vi "SLSC Load EDS Configuration.vi"(0 "selected path":path, 11 "error in (no error)":errorcluster) -> (1 "Type of file":i32(ring) items=["Not a Valid File", "SLSC Capability File", "SLSC EDS Configuration"], 3 "Loop rate":u32, 4 "SLSC EDS module out":T2, 6 "Enable Channels":string[](array[string]), 8 "Custom Device Name":string, 10 "Has capability?":bool, 12 "Apply Default":bool, 13 "Custom Device Description":string, 14 "Apply Reset":bool, 15 "error out":errorcluster)   [LabVIEW 2020, in "SLSC EDS System Explorer.lvlib"]
uses:
  System Explorer/SLSC EDS System Explorer.lvlib
  SLSC EDS API/JSON parsing/EDSjsonStructure.ctl
  SLSC EDS API/JSON parsing/enum.ctl
  SLSC EDS API/JSON parsing/property.ctl
  SLSC EDS API/JSON parsing/command.ctl
  SLSC EDS API/JSON parsing/scale.ctl
  SLSC EDS API/JSON parsing/physicalChannel.ctl
  SLSC EDS API/JSON parsing/register.ctl
  SLSC EDS API/JSON parsing/EDS_Custom_Device_Structure.ctl
  <vilib>/addons/_JKI.lib/Serialization/JSON/JKI JSON Serialization.lvlib
panel:
  out "text":string
  in  "Value":T1
  # "not working\nregisterMap->registers->initialValue"
  # "not working\nregisterMap->registers->initialValue"
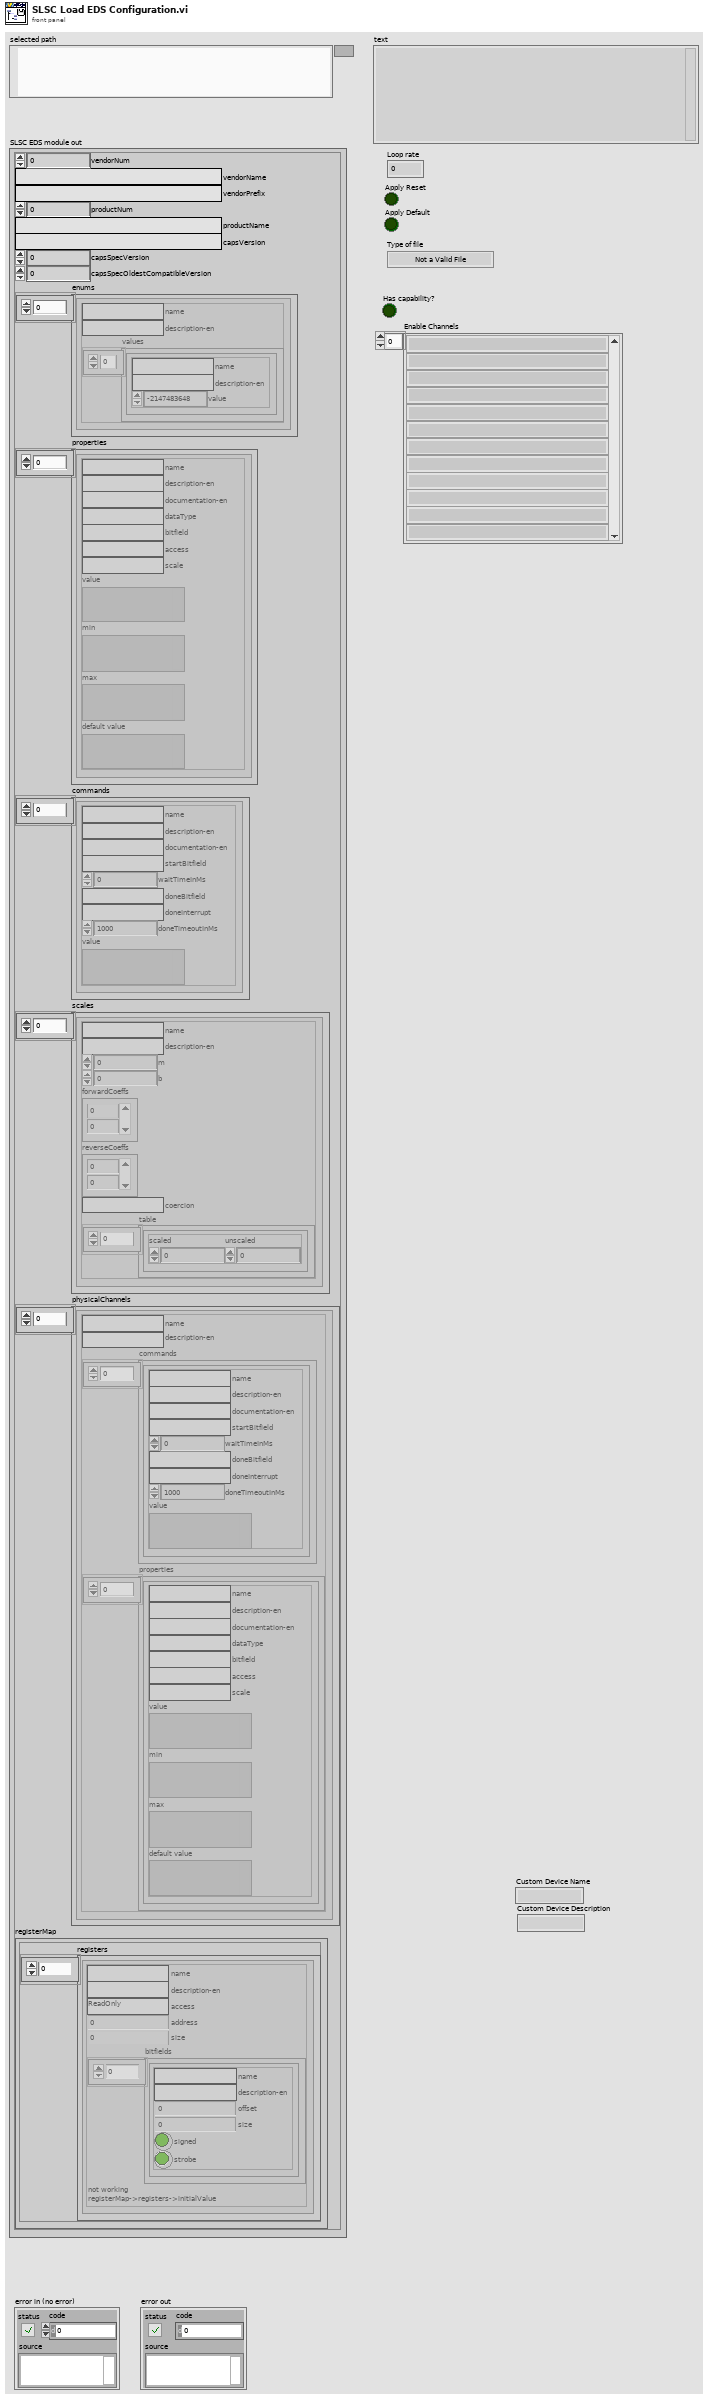
[diagram p1: front panel]
types:
  T1 = typedef "EDS_Custom_Device_Structure.ctl" = cluster{"SLSC EDS module out":T2, "Custom Device Name":string, "TreeItem Channels":string[], "Apply Default":bool, "Apply Reset":bool, "Loop rate":u32, "Custom Device Description":string}
  T2 = typedef "EDSjsonStructure.ctl" = cluster{"vendorNum":u32, "vendorName":string, "vendorPrefix":string, "productNum":u32, "productName":string, "capsVersion":string, "capsSpecVersion":u32, "capsSpecOldestCompatibleVersion":u32, "enums":T3[], "properties":T4[], "commands":T5[], "scales":T6[], "physicalChannels":T7[], "registerMap":cluster{"registers":T8[]}}
  T3 = typedef "enum.ctl" = cluster{"name":string, "description-en":string, "values":cluster{"name":string, "description-en":string, "value":i32}[]}
  T4 = typedef "property.ctl" = cluster{"name":string, "description-en":string, "documentation-en":string, "dataType":string, "bitfield":string, "access":string, "scale":string, "value":variant, "min":variant, "max":variant, "default value":variant}
  T5 = typedef "command.ctl" = cluster{"name":string, "description-en":string, "documentation-en":string, "startBitfield":string, "waitTimeInMs":i32, "doneBitfield":string, "doneInterrupt":string, "doneTimeoutInMs":i32, "value":variant}
  T6 = typedef "scale.ctl" = cluster{"name":string, "description-en":string, "m":dbl, "b":dbl, "forwardCoeffs":dbl[], "reverseCoeffs":dbl[], "coercion":string, "table":cluster{"scaled":dbl, "unscaled":dbl}[]}
  T7 = typedef "physicalChannel.ctl" = cluster{"name":string, "description-en":string, "commands":T5[], "properties":T4[]}
  T8 = typedef "register.ctl" = cluster{"name":string, "description-en":string, "access":string, "address":u32, "size":u32, "bitfields":cluster{"name":string, "description-en":string, "offset":u32, "size":u32, "signed":bool, "strobe":bool}[]}
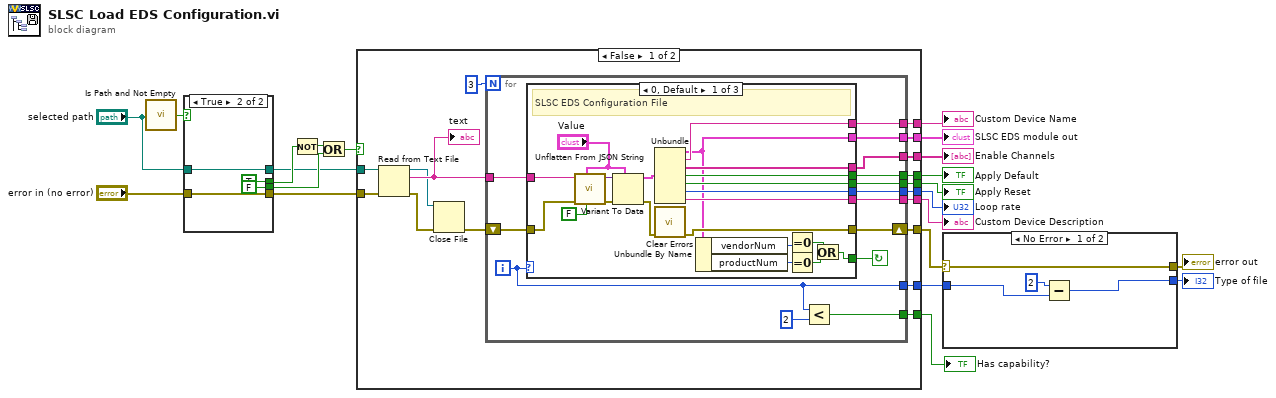
[diagram p0: block diagram]
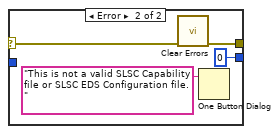
[diagram p2: hidden frame]
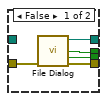
[diagram p3: hidden frame]
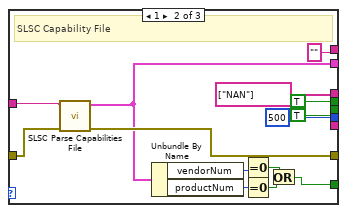
[diagram p4: hidden frame]
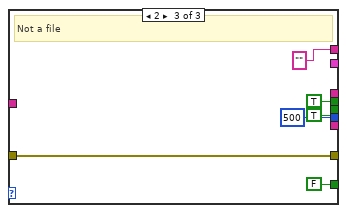
[diagram p5: hidden frame]
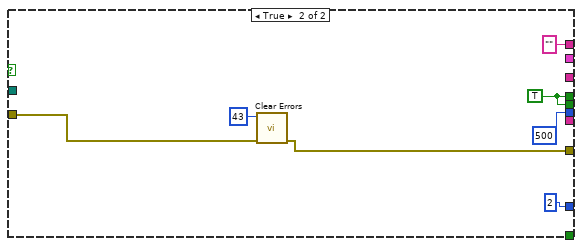
[diagram p6: hidden frame]
diagram:
  n1 = call <vilib>:"Is Path and Not Empty.vi"("path"="selected path") -> ("Is Path and Not Empty?"=w10:bool)  [unwired: 4 in]
  n2 = case shown="True" w10 {
    tunnel: [w26 TRUE ("exists")] -> w17
    tunnel: [w25 FALSE ("cancelled")] -> w15
    tunnel: "error in (no error)" -> [w24 w29]
    tunnel: [w23 w29] -> w13
    tunnel: [w22 w30] -> w12
    tunnel: "selected path" -> [_ w30]
    frame False {
      n3 = call "File Dialog"("error in"=w24) -> ("selected path"=w22:path, "exists"=w26:bool, "cancelled"=w25:bool, "error out"=w23:errorcluster)  [unwired: 11 in]
    }
    frame True {
    }
  }
  n4 = Not(x=w17) -> (.not. x?=w16:bool)
  n5 = Or(x=w16, y=w15) -> (x .or. y?=w11:bool)
  n6 = case shown="False" w11 {
    tunnel: [w47 _] -> w21
    tunnel: [w46 _] -> w20
    tunnel: [w44 w109] -> w2
    tunnel: [w43 w109] -> w1
    tunnel: [w42 u32 500 ("Loop rate")] -> w19
    tunnel: [w40 _] -> w18
    tunnel: [w39 w105] -> w8
    tunnel: w13 -> [w35 w106]
    tunnel: w12 -> [w34 _]
    tunnel: [w33 2] -> w6
    tunnel: [w32 "" ("Custom Device Name")] -> w4
    tunnel: [w31 _] -> w3
    frame False {
      n7 = Read from Text File(file (use dialog)=w34, error in=w35) -> (refnum out=w37:refnum<file>, text=w45:string, error out=w38:errorcluster)  [unwired: 2 in, 1 out]
      "text" <- w45
      n8 = Close File(refnum=w37, error in=w38) -> (error out=w36:errorcluster)  [unwired: 1 out]
      n9 = for {
        N: 3 -> [_]
        tunnel: [w60] -> w47
        tunnel: [w59] -> w46
        tunnel: w45 -> [w57]
        tunnel: [w56] -> w44
        tunnel: [w55] -> w43
        tunnel: [w54] -> w42
        shift-right: [w58] -> w39
        shift-left: w36 -> [w61]
        tunnel: [w51] -> w40
        tunnel: [w50] -> w33
        tunnel: [w49] -> w32
        tunnel: [w48] -> w31
        i -> [w50]
        stop <- w53 continue-if-true
        n10 = case shown="0, Default" w50 {
          tunnel: w61 -> [w82 w86 w99]
          tunnel: [w68 string[] ["NAN"] ("TreeItem Channels") _] -> w60
          tunnel: [w62 w84 _] -> w59
          tunnel: [w69 w85 w99] -> w58
          tunnel: w57 -> [w80 w87 _]
          tunnel: [w67 TRUE ("Apply Reset") TRUE ("Apply Reset")] -> w56
          tunnel: [w66 TRUE ("Apply Default") TRUE ("Apply Default")] -> w55
          tunnel: [w65 u32 500 ("Loop rate") u32 500 ("Loop rate")] -> w54
          tunnel: [w72 w89 FALSE] -> w53
          tunnel: [w63 "" ("Custom Device Name") "" ("Custom Device Name")] -> w49
          tunnel: [w64 _ _] -> w48
          frame 0, Default {
            # "SLSC EDS Configuration File"
            n11 = call <vilib>:"Unflatten From JSON String.vi"("Nulls as Defaults (F)"=FALSE, "Type and Defaults"="Value", "error in (no error)"=w82, "JSON String"=w80) -> ("error out"=w77:errorcluster, "Variant"=w78:variant)  [unwired: 6 in]
            n12 = Variant To Data(error in=w77, type="Value", Variant=w78) -> (data=w81:T1, error out=w70:errorcluster)
            n13 = Unbundle(w81) -> ("SLSC EDS module out"=w62:T2, "Custom Device Name"=w63:string, "TreeItem Channels"=w68:string[], "Apply Default"=w67:bool, "Apply Reset"=w66:bool, "Loop rate"=w65:u32, "Custom Device Description"=w64:string)
            n14 = call <vilib>:"Clear Errors.vi"("error in (no error)"=w70) -> ("error out"=w69:errorcluster)  [unwired: 5 in, 1 out]
            n15 = Unbundle By Name(w62) -> ("vendorNum"=w74:u32, "productNum"=w73:u32)
            n16 = Equal To 0?(x=w74) -> (x = 0?=w75:bool)
            n17 = Equal To 0?(x=w73) -> (x = 0?=w71:bool)
            n18 = Or(x=w75, y=w71) -> (x .or. y?=w72:bool)
          }
          frame 1 {
            # "SLSC Capability File"
            n19 = call "SLSC Parse Capabilities File.vi"("error in"=w86, "module capabilities JSON string"=w87) -> ("error out"=w85:errorcluster, "SLSC EDS module"=w84:T2)  [unwired: 7 in, 1 out]
            n20 = Unbundle By Name(w84) -> ("vendorNum"=w92:u32, "productNum"=w91:u32)
            n21 = Equal To 0?(x=w92) -> (x = 0?=w93:bool)
            n22 = Equal To 0?(x=w91) -> (x = 0?=w90:bool)
            n23 = Or(x=w93, y=w90) -> (x .or. y?=w89:bool)
          }
          frame 2 {
            # "Not a file"
          }
        }
        n24 = Less?(x=w50, y=2) -> (x < y?=w51:bool)
      }
    }
    frame True {
      w109 = TRUE ("Apply Reset")
      n25 = call <vilib>:"Clear Errors.vi"("error in (no error)"=w106, "specific error code to clear (0: all)"=43) -> ("error out"=w105:errorcluster)  [unwired: 4 in, 1 out]
    }
  }
  "Enable Channels" <- w21
  "SLSC EDS module out" <- w20
  "Apply Reset" <- w1
  "Apply Default" <- w2
  "Loop rate" <- w19
  "Has capability?" <- w18
  "Custom Device Name" <- w4
  "Custom Device Description" <- w3
  n26 = case shown="No Error" w8 {
    selector: w8 -> [w113 w115]
    tunnel: [w113 w116] -> w7
    tunnel: [w111 0] -> w5
    tunnel: w6 -> [w112 _]
    frame No Error {
      n27 = Subtract(x=2, y=w112) -> (x-y=w111:i32)
    }
    frame Error {
      n28 = call <vilib>:"Clear Errors.vi"("error in (no error)"=w115) -> ("error out"=w116:errorcluster)  [unwired: 5 in, 1 out]
      n29 = One Button Dialog(message="This is not a valid SLSC Capability file or SLSC EDS Configuration file.") -> ()  [unwired: 1 in, 1 out]
    }
  }
  "error out" <- w7
  "Type of file" <- w5
